vi "destroy.vi"(8 "error in":errorcluster, 11 "websocket user plugin in":refnum<class "websocket user plugin.lvclass">) -> (0 "error out":errorcluster)   [LabVIEW 2016, in "websocket user plugin.lvclass"]
uses:
  websocket user plugin.lvclass
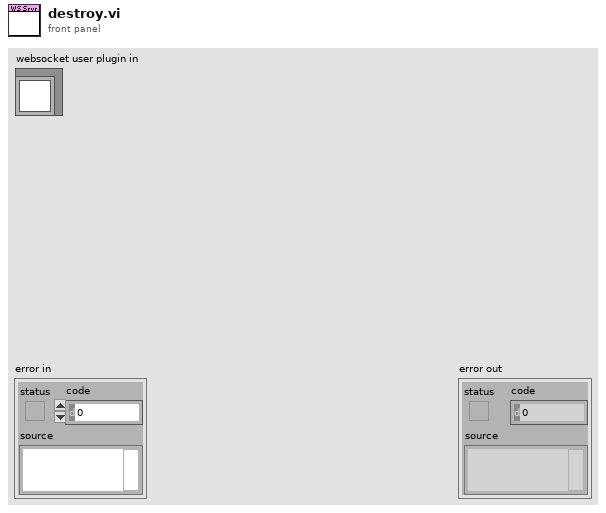
[diagram p1: front panel]
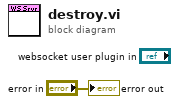
[diagram p0: block diagram]
diagram:
  "error out" <- "error in"
